vi "TimedOut.vi"(8 "WaitTime":dbl, 9 "MotorPower":dbl, 10 "Button":bool, 11 "MotorIn":dbl) -> (0 "Completed?":bool, 3 "MotorOut":dbl)   [LabVIEW 2015]
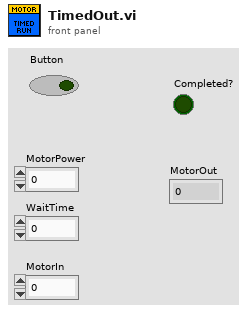
[diagram p1: front panel]
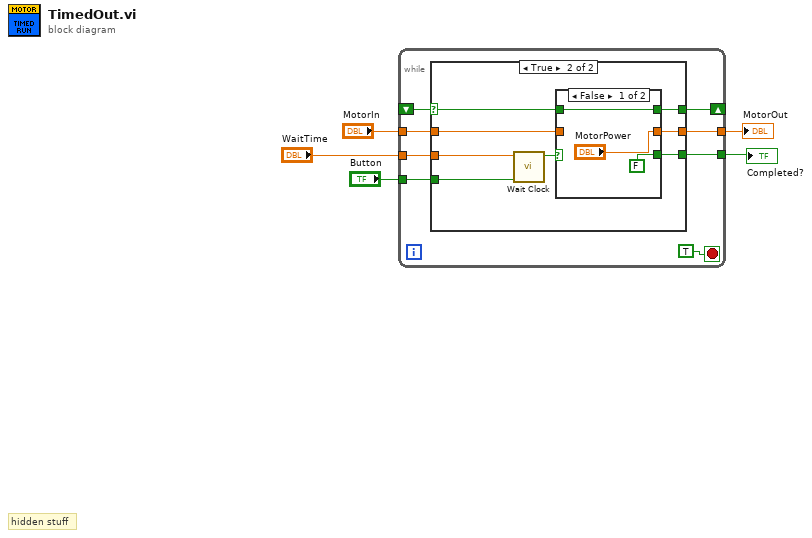
[diagram p0: block diagram]
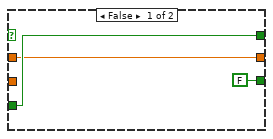
[diagram p2: hidden frame]
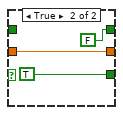
[diagram p3: hidden frame]
diagram:
  # "hidden stuff"
  n1 = while {
    tunnel: "Button" -> [w8]
    shift-right: [w13] -> _
    shift-left: _ -> [w12]
    tunnel: [w11] -> w4
    tunnel: "MotorIn" -> [w10]
    tunnel: "WaitTime" -> [w7]
    tunnel: [w6] -> w1
    stop <- TRUE stop-if-true
    n2 = case shown="True" w12 {
      selector: w12 -> [_ w20]
      tunnel: [w16 w19] -> w13
      tunnel: w8 -> [w16 w23]
      tunnel: [w15 w22] -> w11
      tunnel: w10 -> [w15 w21]
      tunnel: w7 -> [_ w18]
      tunnel: [FALSE ("Completed?") w17] -> w6
      frame False {
      }
      frame True {
        n3 = call "Wait Clock.vi"("First Time?"=w23, "Target Time"=w18) -> ("Completed"=w24:bool)  [unwired: 9 in]
        n4 = case shown="False" w24 {
          tunnel: ["MotorPower" w30] -> w22
          tunnel: w21 -> [_ w30]
          tunnel: w20 -> [w26 _]
          tunnel: [w26 FALSE] -> w19
          tunnel: [FALSE ("Completed?") TRUE ("Completed?")] -> w17
          frame False {
          }
          frame True {
          }
        }
      }
    }
  }
  "MotorOut" <- w4
  "Completed?" <- w1
